vi "Main.vi"() -> ()   [LabVIEW 2019]
doc: "The myRIO Project template acquires acceleration data from the onboard accelerometer and displays the changes of acceleration values in a waveform chart."
uses:
  <vilib>/myRIO/Instrument Drivers/Onboard Devices/Accelerometer/typedefs/Accelerometer Reference.ctl
  <vilib>/myRIO/Common/Instrument Driver Framework/Utilities/typedefs/myRIO Generic Hardware Reference.ctl
  <vilib>/myRIO/Common/Instrument Driver Framework/Utilities/typedefs/Hardware Version Enum.ctl
  <vilib>/myRIO/Common/Instrument Driver Framework/Utilities/typedefs/myRIO v1.0 Reference.ctl
  <vilib>/myRIO/Common/Instrument Driver Framework/Utilities/typedefs/Generic FPGA Reference.ctl
  <vilib>/myRIO/Common/Instrument Driver Framework/myRIO v1.0/Accelerometer/typedefs/Accelerometer Channels List.ctl
  <vilib>/myRIO/Common/Instrument Driver Framework/myRIO v1.0/Accelerometer/typedefs/Accelerometer Channels Enum.ctl
  <vilib>/userDefined/High Color/nirio_resource_hc.ctl
  <vilib>/myRIO/Common/Instrument Driver Framework/Utilities/vis/Is FPGA Ref Available.vi
  <vilib>/myRIO/Common/Instrument Driver Framework/myRIO v1.0/Accelerometer/vis/myRIO v1.1 Open Accelerometer.vi
  <vilib>/myRIO/Instrument Drivers/Onboard Devices/Accelerometer/vis/Read.vi
  <vilib>/myRIO/Common/Instrument Driver Framework/myRIO v1.0/PWM/vis/myRIO v1.1 Open PWM.vi
  <vilib>/myRIO/Common/Instrument Driver Framework/Utilities/vis/Validate Channels.vi
  <vilib>/myRIO/Common/Instrument Driver Framework/myRIO v1.0/Accelerometer/vis/myRIO v1.0 Reserve Accelerometer.vi
  <vilib>/myRIO/Common/Instrument Driver Framework/myRIO v1.0/UART/vis/myRIO v1.0 Close UART.vi
  <vilib>/myRIO/Common/Instrument Driver Framework/myRIO v1.0/PWM/vis/myRIO v1.0 Reserve PWM.vi
  <vilib>/myRIO/Common/Instrument Driver Framework/myRIO v1.0/Resource Manager/vis/myRIO v1.0 Reserve Channel List.vi
  <vilib>/myRIO/Common/Instrument Driver Framework/myRIO v1.0/Accelerometer/vis/myRIO v1.0 Build MUX Configuration Accelerometer.vi
  <vilib>/myRIO/Common/Instrument Driver Framework/myRIO v1.0/PWM/vis/myRIO v1.0 Build MUX Configuration PWM.vi
  <vilib>/myRIO/Common/Instrument Driver Framework/myRIO v1.0/Resource Manager/vis/myRIO v1.0 Reserve Channel.vi
  <vilib>/myRIO/Common/Instrument Driver Framework/myRIO v1.0/Resource Manager/vis/myRIO v1.0 Unreserve Channel.vi
  <vilib>/myRIO/Common/Instrument Driver Framework/myRIO v1.0/Resource Manager/vis/myRIO v1.0 Create Configuration List.vi
  <vilib>/myRIO/Common/Instrument Driver Framework/myRIO v1.0/Resource Manager/vis/myRIO v1.0 Build Mutex Name.vi
  <vilib>/Utility/VariantDataType/GetNumericInfo.vi
  <vilib>/Utility/error.llb/Error Cluster From Error Code.vi
  <vilib>/myRIO/Common/Instrument Driver Framework/myRIO v1.0/myRIO v1.1 Open.vi
  <vilib>/myRIO/Common/Instrument Driver Framework/Utilities/vis/IO Manager.vi
  <vilib>/myRIO/Common/Instrument Driver Framework/Utilities/vis/Configuration Manager.vi
  <vilib>/myRIO/Common/Instrument Driver Framework/myRIO v1.0/Resource Manager/vis/myRIO v1.0 Configure IO.vi
  <vilib>/myRIO/Common/Instrument Driver Framework/myRIO v1.0/myRIO v1.0 Close.vi
  <vilib>/myRIO/Common/Instrument Driver Framework/myRIO v1.0/Accelerometer/vis/myRIO v1.0 Get Scaling Constant Accelerometer.vi
  <vilib>/myRIO/Common/Instrument Driver Framework/myRIO v1.0/Accelerometer/vis/myRIO v1.0 Read Accelerometer.vi
  <vilib>/myRIO/Common/Instrument Driver Framework/myRIO v1.0/PWM/vis/myRIO v1.0 Write PWM.vi
  <vilib>/myRIO/Common/Instrument Driver Framework/Utilities/vis/FPGA Ref Manager.vi
  <vilib>/myRIO/Common/Instrument Driver Framework/myRIO v1.0/myRIO v1.0 Reset FPGA.vi
  <vilib>/myRIO/Common/Instrument Driver Framework/myRIO v1.0/IRQ/vis/myRIO v1.0 IRQ Info FGV.vi
  <vilib>/myRIO/Common/Instrument Driver Framework/myRIO v1.0/IRQ/vis/myRIO v1.0 Timer IRQ Info FGV.vi
  <vilib>/myRIO/Common/Instrument Driver Framework/myRIO v1.0/IRQ/vis/myRIO v1.0 ISR Agent.vi
  <vilib>/myRIO/Instrument Drivers/Utilities/vis/Reset Index.vi
  <vilib>/myRIO/Common/Instrument Driver Framework/myRIO v1.0/Resource Manager/vis/myRIO v1.0 Block Write Resource Manager.vi
  <vilib>/myRIO/Express VI/Onboard Devices/Accelerometer/Accelerometer Express VI.xnode
  <vilib>/myRIO/Instrument Drivers/Onboard Devices/Accelerometer/vis/myRIO Accelerometer Open.xnode
  <vilib>/myRIO/Instrument Drivers/Utilities/Utilities.lvlib
  <vilib>/myRIO/Instrument Drivers/Onboard Devices/Accelerometer/Accelerometer.lvlib
  <vilib>/myRIO/Instrument Drivers/Onboard IO/PWM/PWM.lvlib
panel:
  out "Y-Axis":dbl
  in  "[ESC]":bool
  out "pulse width [ms]":dbl=1.5
  out "duty cycle [%]":dbl
  in  "freq [Hz]":dbl(slide)=50.0 scale=0.0..200.0
  out "Acceleration":T1(graph)
  out "error out":errorcluster
  in  "Stop":bool
  # "Overview: The myRIO Project template acquires acceleration data from the onboard accelerometer and displays the changes of acceleration values in a waveform chart.\nInstructions:\n1. Check the myRIO target IP address in the project and make sure the target IP address is correct. \n2. Run this VI."
  # "Servo Iris Mechanism"
  # "TUTUP"
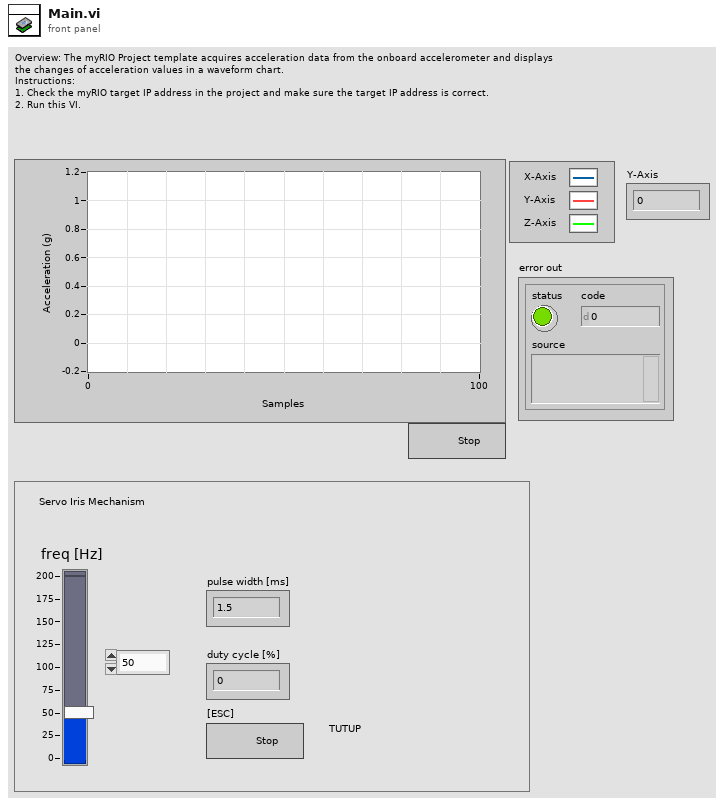
[diagram p1: front panel]
types:
  T1 = cluster{"X-Axis":dbl, "Y-Axis":dbl, "Z-Axis":dbl}
  T2 = typedef "Accelerometer.lvlib/Accelerometer Reference.ctl" = cluster{"myRIO Reference":T3, "Accelerometer Channels List":T7, "LSB Weight":dbl}
  T3 = typedef "myRIO Generic Hardware Reference.ctl" = cluster{"myRIO Model":T4, "myRIO Hardware Reference":T5}
  T4 = typedef "Hardware Version Enum.ctl" = enum16{"Unknown", "myRIO-1900", "myRIO-1950", "roboRIO", "NI ELVIS RIO CM", "ELVIS III"}
  T5 = typedef "myRIO v1.0 Reference.ctl" = cluster{"Generic FPGA Reference":T6, "Allow multiple opens":bool}
  T6 = typedef "Generic FPGA Reference.ctl" = refnum<k20>
  T7 = typedef "Accelerometer Channels List.ctl" = T8[]
  T8 = typedef "Accelerometer Channels Enum.ctl" = enum16{"Not Connected", "X-Axis", "Y-Axis", "Z-Axis"}
  T9 = typedef "nirio_resource_hc.ctl" = tag
  T10 = typedef "PWM.lvlib/PWM Reference.ctl" = cluster{"myRIO Reference":T3, "PWM Channels Enum":T11, "PWM Configuration":T12}
  T11 = typedef "PWM Channels Enum.ctl" = enum16{"Not Connected", "C/PWM0", "C/PWM1", "A/PWM0", "A/PWM1", "A/PWM2", "A/PWM3", "A/PWM4", "A/PWM5", "A/PWM6", "A/PWM7", "A/PWM8", "A/PWM9", "A/PWM10", "A/PWM11", "A/PWM12", "A/PWM13", "A/PWM14", "A/PWM15", "A/PWM16", "A/PWM17", "A/PWM18", "A/PWM19", "B/PWM0", "B/PWM1", "B/PWM2", "B/PWM3", "B/PWM4", "B/PWM5", "B/PWM6", "B/PWM7", "B/PWM8", "B/PWM9", "B/PWM10", "B/PWM11", "B/PWM12", "B/PWM13", "B/PWM14", "B/PWM15", "B/PWM16", "B/PWM17", "B/PWM18", "B/PWM19", "PWM/PWM0", "PWM/PWM1", "PWM/PWM2", "PWM/PWM3", "PWM/PWM4", "PWM/PWM5", "PWM/PWM6", "PWM/PWM7", "PWM/PWM8", "PWM/PWM9"}
  T12 = typedef "PWM.lvlib/PWM Configuration.ctl" = cluster{"Frequency":dbl, "Duty Cycle":dbl}
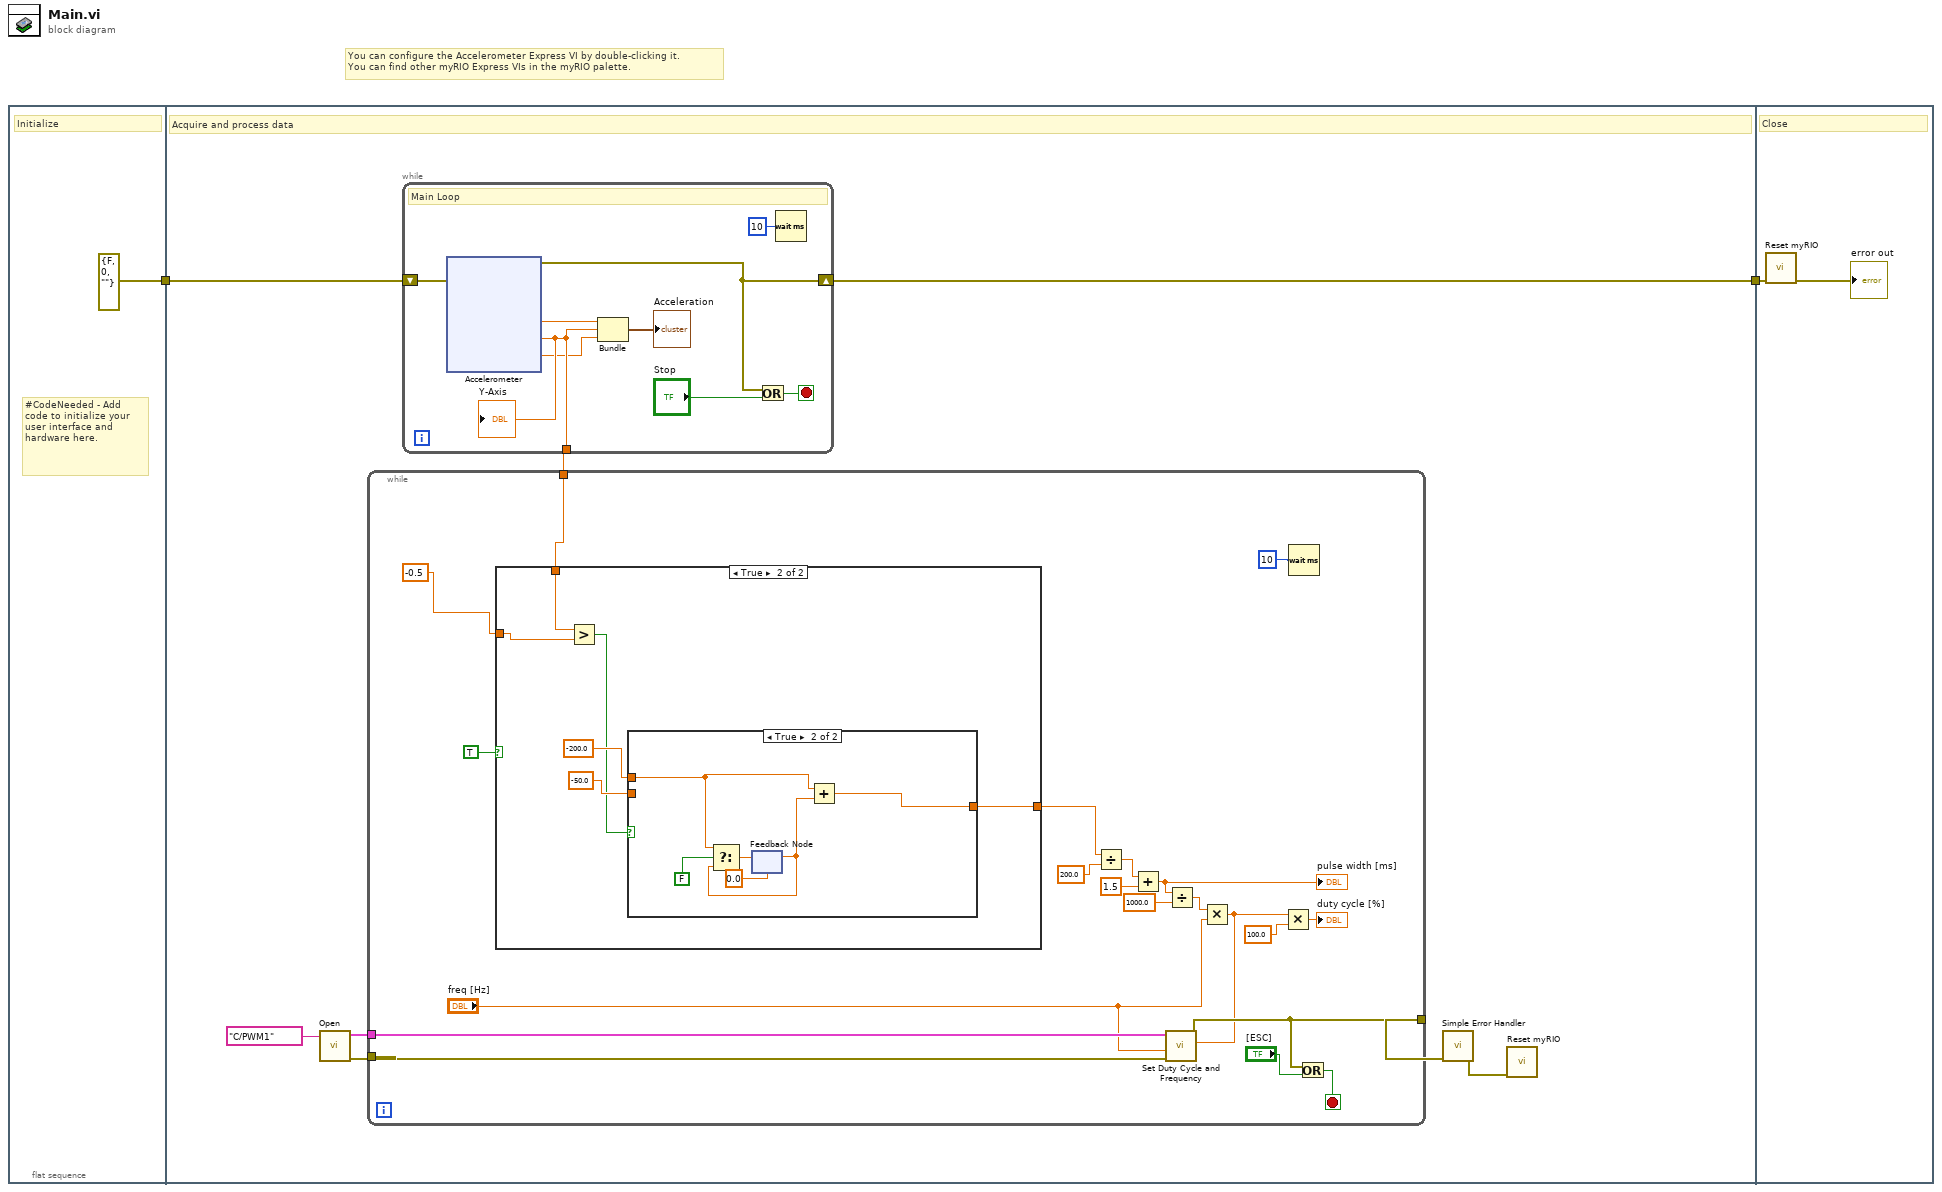
[diagram p0: block diagram]
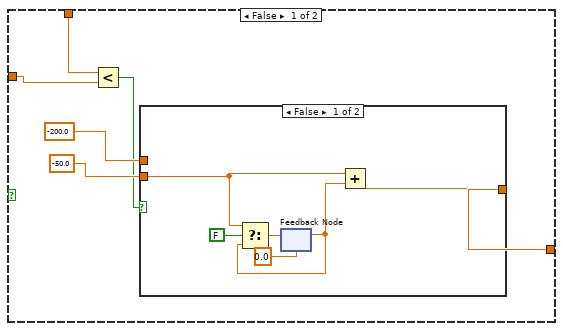
[diagram p2: hidden frame]
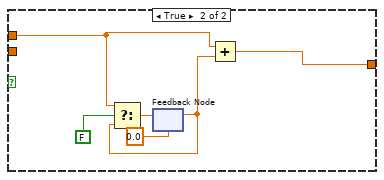
[diagram p3: hidden frame]
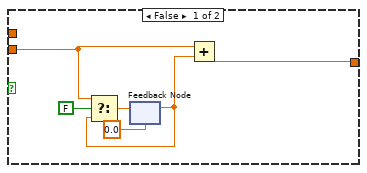
[diagram p4: hidden frame]
diagram:
  # "You can configure the Accelerometer Express VI by double-clicking it.\nYou can find other myRIO Express VIs in the myRIO palette."
  n1 = flat-sequence {
    tunnel: [errorcluster {"status"=FALSE, "code"=0, "source"=""} ("error in (no error)")] -> w2
    tunnel: w2 -> [w11]
    tunnel: [w10] -> w1
    tunnel: w1 -> [w117]
    frame #0 {
      # "#CodeNeeded - Add code to initialize your user interface and hardware here."
      # "Initialize"
    }
    frame #1 {
      # "Acquire and process data"
      n2 = call <vilib>:"Open.vi"("Channel Name"=tag "C/PWM1") -> ("error out"=w7:errorcluster, "PWM Ref Out"=w8:T10)  [unwired: 9 in]
      n3 = while {
        shift-right: [w71] -> w10
        shift-left: w11 -> [w72]
        tunnel: [w70] -> w4
        stop <- w75 stop-if-true
        # "Main Loop"
        n4 = xnode "Accelerometer"("error in (no error)"=w72) -> ("X-Axis"=w68:dbl, "Y-Axis"=w70:dbl, "Z-Axis"=w69:dbl, "error out"=w71:errorcluster)
        "Y-Axis" <- w70
        n5 = Bundle("X-Axis"=w68, "Y-Axis"=w70, "Z-Axis"=w69) -> (→"Acceleration":T1)  [unwired: 1 in]
        n6 = Or(x=w71, y="Stop") -> (x .or. y?=w75:bool)
        n7 = Wait (ms)(milliseconds to wait=u32 10) -> ()  [unwired: 1 out]
      }
      n8 = while {
        tunnel: w8 -> [w29]
        tunnel: w7 -> [w28]
        tunnel: [w27] -> w6
        tunnel: w4 -> [w14]
        stop <- w31 stop-if-true
        n9 = case shown="True" TRUE {
          tunnel: [w35 w53] -> w15
          tunnel: w14 -> [w34 w52]
          tunnel: -0.5 -> [w33 w51]
          frame False {
            n10 = Less?(x=w34, y=w33) -> (x < y?=w32:bool)
            n11 = case shown="False" w32 {
              tunnel: -200.0 ("x") -> [_ w46]
              tunnel: -50.0 ("x") -> [w40 _]
              tunnel: [w38 w45] -> w35
              frame False {
                n12 = feedback #1(0.0 ("position [%FS]")) -> (w39:dbl)
                n13 = Select(t=w40, s=FALSE, f=w39) -> (s? t:f=w43:dbl)
                n14 = feedback-in #1(w43) -> ()
                n15 = Add(x=w40, y=w39) -> (x+y=w38:dbl)
              }
              frame True {
                n16 = feedback #2(0.0 ("position [%FS]")) -> (w44:dbl)
                n17 = Select(t=w46, s=FALSE, f=w44) -> (s? t:f=w49:dbl)
                n18 = feedback-in #2(w49) -> ()
                n19 = Add(x=w46, y=w44) -> (x+y=w45:dbl)
              }
            }
          }
          frame True {
            n20 = Greater?(x=w52, y=w51) -> (0:w50:bool)
            n21 = case shown="True" w50 {
              tunnel: -200.0 ("x") -> [_ w64]
              tunnel: -50.0 ("x") -> [w58 _]
              tunnel: [w56 w63] -> w53
              frame False {
                n22 = feedback #3(0.0 ("position [%FS]")) -> (w57:dbl)
                n23 = Select(t=w58, s=FALSE, f=w57) -> (s? t:f=w61:dbl)
                n24 = feedback-in #3(w61) -> ()
                n25 = Add(x=w58, y=w57) -> (x+y=w56:dbl)
              }
              frame True {
                n26 = feedback #4(0.0 ("position [%FS]")) -> (w62:dbl)
                n27 = Select(t=w64, s=FALSE, f=w62) -> (s? t:f=w67:dbl)
                n28 = feedback-in #4(w67) -> ()
                n29 = Add(x=w64, y=w62) -> (x+y=w63:dbl)
              }
            }
          }
        }
        n30 = Divide(x=w15, y=200.0) -> (x/y=w22:dbl)
        n31 = Add(x=w22, y=1.5) -> (x+y=w20:dbl)
        "pulse width [ms]" <- w20
        n32 = Divide(x=w20, y=1000.0) -> (x/y=w18:dbl)
        n33 = Multiply(x=w18, y="freq [Hz]") -> (x*y=w26:dbl)
        n34 = call <vilib>:"Set Duty Cycle and Frequency.vi"("error in (no error)"=w28, "Frequency [Hz]"="freq [Hz]", "Duty Cycle"=w26, "PWM Ref In"=w29) -> ("error out"=w27:errorcluster)  [unwired: 5 in, 1 out]
        n35 = Multiply(x=w26, y=100.0) -> (x*y=→"duty cycle [%]":dbl)
        n36 = Wait (ms)(milliseconds to wait=u32 10) -> ()  [unwired: 1 out]
        n37 = Or(x=w27, y="[ESC]") -> (x .or. y?=w31:bool)
      }
      n38 = call <vilib>:"Simple Error Handler.vi"("error in (no error)"=w6) -> ("error out"=w9:errorcluster)  [unwired: 4 in, 4 out]
      n39 = call <vilib>:"Reset myRIO.vi"("error in (no error)"=w9) -> ()  [unwired: 10 in, 1 out]
    }
    frame #2 {
      # "Close"
      n40 = call <vilib>:"Reset myRIO.vi"("error in (no error)"=w117) -> ("error out"=→"error out":errorcluster)  [unwired: 10 in]
    }
  }
